vi "write_sample_results_files.vi"(8 "Error In":errorcluster, 9 "Sample Results":T1, 10 "Sample":string, 11 "File Path":path) -> (0 "Error Out":errorcluster)   [LabVIEW 2019]
uses:
  sample_results_cluster_typedef.ctl
  parameters_cluster_typedef.ctl
  writeable_section_parameters_cluster_typedef.ctl
  grain_results_cluster_typedef.ctl
panel:
  out "Exists?":bool
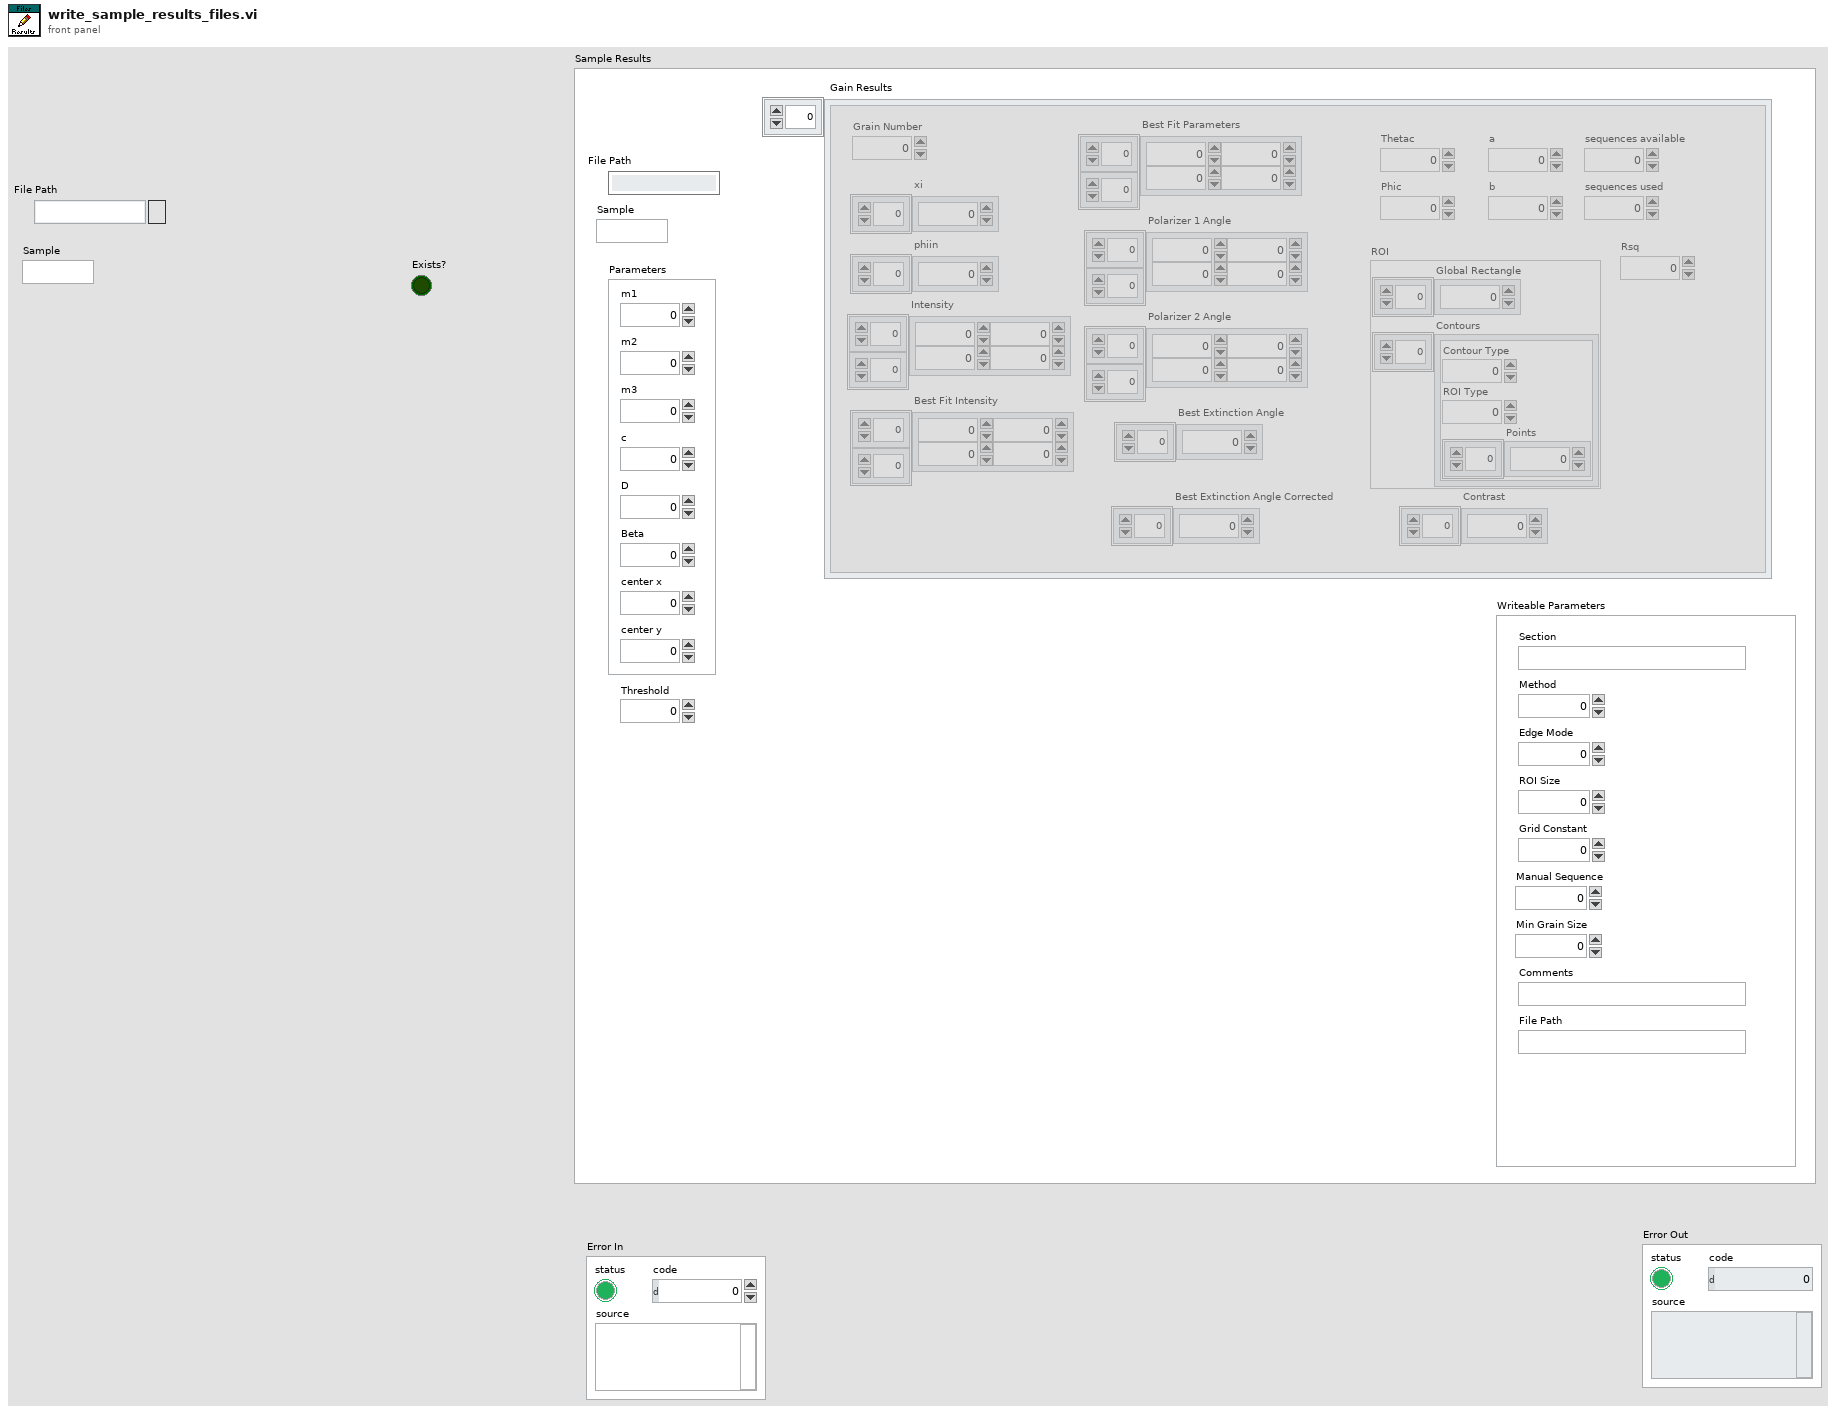
[diagram p1: front panel]
types:
  T1 = typedef "sample_results_cluster_typedef.ctl" = cluster{"File Path":string, "Sample":string, "Threshold":dbl, "Parameters":T2, "Writeable Parameters":T3, "Gain Results":T4[]}
  T2 = typedef "parameters_cluster_typedef.ctl" = cluster{"m1":dbl, "m2":dbl, "m3":dbl, "c":dbl, "D":dbl, "Beta":dbl, "center x":dbl, "center y":dbl}
  T3 = typedef "writeable_section_parameters_cluster_typedef.ctl" = cluster{"Section":string, "Method":i32, "Edge Mode":i32, "Grid Constant":i32, "Manual Sequence":i32, "ROI Size":i32, "Min Grain Size":dbl, "Comments":string, "File Path":string}
  T4 = typedef "grain_results_cluster_typedef.ctl" = cluster{"Grain Number":i32, "xi":dbl[], "phiin":dbl[], "Intensity":dbl[][], "Best Fit Intensity":dbl[][], "Best Fit Parameters":dbl[][], "Polarizer 1 Angle":dbl[][], "Polarizer 2 Angle":dbl[][], "Best Extinction Angle":dbl[], "Best Extinction Angle Corrected":dbl[], "Thetac":dbl, "Phic":dbl, "ROI":cluster{"Global Rectangle":i32[], "Contours":cluster{"Contour Type":u32, "ROI Type":u32, "Points":i32[]}[]}, "a":dbl, "b":dbl, "sequences available":dbl, "sequences used":dbl, "Contrast":dbl[], "Rsq":dbl}
  T5 = enum16{"open", "replace", "create", "open or create", "replace or create", "replace or create with confirmation"}
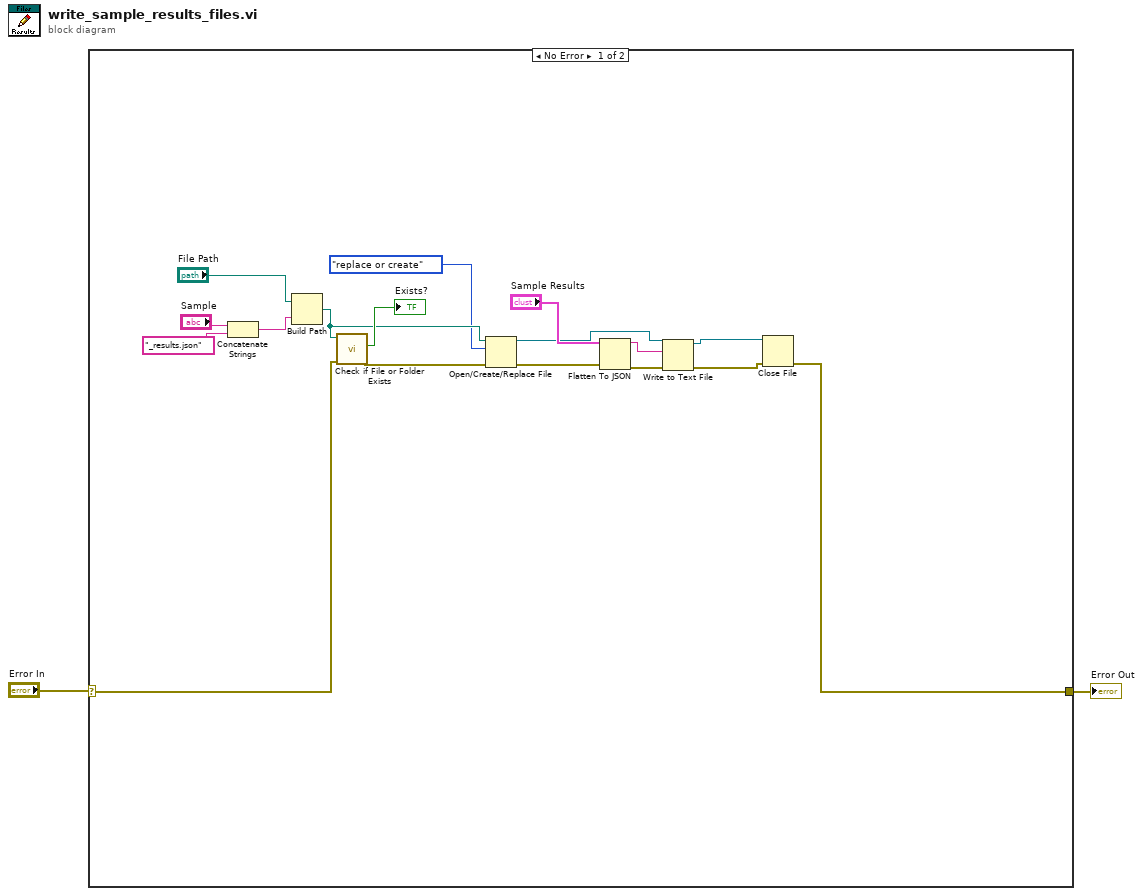
[diagram p0: block diagram]
diagram:
  n1 = case shown="No Error" "Error In" {
    selector: "Error In" -> [w14 w20]
    tunnel: [w10 w20] -> w1
    frame No Error {
      n2 = Concatenate Strings("Sample", "_results.json" ("string")) -> (w19:string)
      n3 = Build Path(base path="File Path", name or relative path=w19) -> (appended path=w12:path)
      n4 = call <vilib>:"Check if File or Folder Exists.vi"("error in (no error)"=w14, "path"=w12) -> ("error out"=w13:errorcluster, "file or folder exists?"=→"Exists?":bool)  [unwired: 7 in, 1 out]
      n5 = Open/Create/Replace File(file path (use dialog)=w12, error in=w13, operation (0:open)=T5."replace or create") -> (refnum out=w4:refnum<file>, error out=w3:errorcluster)  [unwired: 3 in, 1 out]
      n6 = Flatten To JSON(anything="Sample Results", error in (no error)=w3) -> (JSON string=w8:string, 11:w5:errorcluster)  [unwired: 1 in]
      n7 = Write to Text File(file (use dialog)=w4, text=w8, error in=w5) -> (refnum out=w7:refnum<file>, error out=w6:errorcluster)  [unwired: 1 in, 1 out]
      n8 = Close File(refnum=w7, error in=w6) -> (error out=w10:errorcluster)  [unwired: 1 out]
    }
    frame Error {
    }
  }
  "Error Out" <- w1
